vi "Calc RMS V and I.vi"(11 "LAB01-1 (GRAPH)":dynamicdata(waveform)) -> (2 "RMS V":dbl, 3 "RMS I":dbl)   [LabVIEW 2017]
doc: "Calculate value of saturated waveform"
uses:
  <vilib>/measure/madcrms.llb/Basic Averaged DC-RMS for N Chan.vi
  <vilib>/measure/NI_MAPro.lvlib
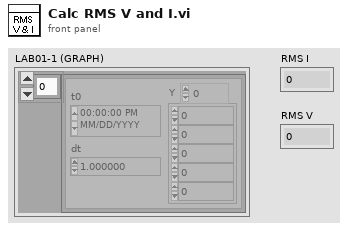
[diagram p1: front panel]
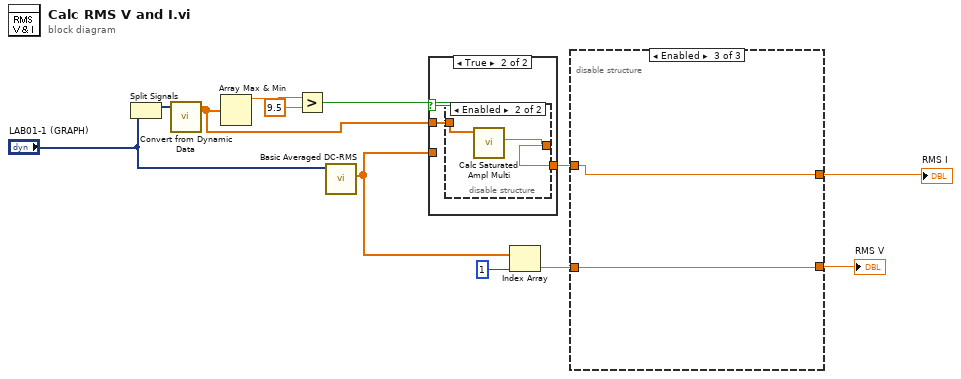
[diagram p0: block diagram]
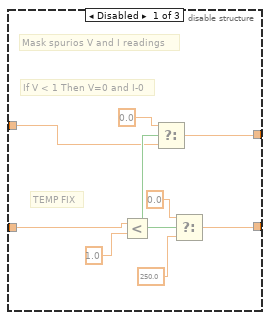
[diagram p2: hidden frame]
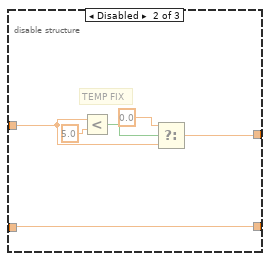
[diagram p3: hidden frame]
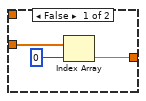
[diagram p4: hidden frame]
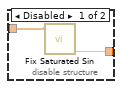
[diagram p5: hidden frame]
diagram:
  n1 = Split Signals("LAB01-1 (GRAPH)") -> (w8:dynamicdata)  [unwired: 2 in, 1 out]
  n2 = call "Convert from Dynamic Data"("Dynamic Data Type"=w8) -> ("Array"=w10:dbl[])  [unwired: 3 in]
  n3 = Array Max & Min(array=w10) -> (max value=w11:dbl)  [unwired: 3 out]
  n4 = Greater?(x=w11, y=9.5) -> (0:w9:bool)
  n5 = call-poly <vilib>:"Basic Averaged DC-RMS.vi"("signals in"="LAB01-1 (GRAPH)") -> ("RMS values"=w6:dbl[])  [unwired: 7 in, 3 out]
  n6 = case shown="True" w9 {
    tunnel: w6 -> [w15 _]
    tunnel: [w13 w16] -> w4
    tunnel: w10 -> [_ w17]
    frame False {
      n7 = Index Array(array=w15, index=0) -> (element=w13:dbl)
    }
    frame True {
      n8 = disable-structure shown="Enabled" {
        disable-tunnel: w17 -> [w19 w21]
        disable-tunnel: [w18 w20] -> w16
        frame Disabled {
          n9 = call "Fix Saturated Sin.vi"("Waveform"=w19) -> ("RMS value"=w18:dbl)  [unwired: 3 in, 7 out]
        }
        frame Enabled {
          n10 = call "Calc Saturated Ampl Multi.vi"("Data"=w21) -> ("mean"=w20:dbl)  [unwired: 6 in, 4 out]
        }
      }
    }
  }
  n11 = Index Array(array=w6, index=1) -> (element=w1:dbl)
  n12 = disable-structure shown="Enabled" {
    disable-tunnel: [w30 w36 w37] -> w5
    disable-tunnel: w4 -> [w24 w34 w37]
    disable-tunnel: [w23 w31 w38] -> w3
    disable-tunnel: w1 -> [w22 w31 w38]
    frame Disabled {
      # "Mask spurios V and I readings"
      # "If V < 1 Then V=0 and I-0"
      # "TEMP FIX"
      n13 = Less?(x=w22, y=1.0) -> (x < y?=w25:bool)
      n14 = Select(t=0.0 ("f"), s=w25, f=w24) -> (s? t:f=w30:dbl)
      n15 = Select(t=0.0, s=w25, f=250.0) -> (s? t:f=w23:dbl)
    }
    frame Disabled {
      # "TEMP FIX"
      n16 = Less?(x=w34, y=5.0) -> (x < y?=w32:bool)
      n17 = Select(t=0.0 ("f"), s=w32, f=w34) -> (s? t:f=w36:dbl)
    }
    frame Enabled {
    }
  }
  "RMS V" <- w3
  "RMS I" <- w5
